vi "E14 BBB Test.vi"(8 "Error In":errorcluster, 10 "Credentials":T1, 11 "SSH Session":refnum<k24>) -> (0 "Error Out":errorcluster, 3 "SSH Session":refnum<k24>)   [LabVIEW 2014, in "LMH-LINX.lvlib"]
uses:
  LMH-LINX.lvlib
  C:/github/makerhub/LINX/LabVIEW/vi.lib/MakerHub/LINX/Private/Utilties/Renci.SshNet.dll
  Renci.SshNet.dll
  <vilib>/MakerHub/Toolbox/LMH-Toolbox.lvlib
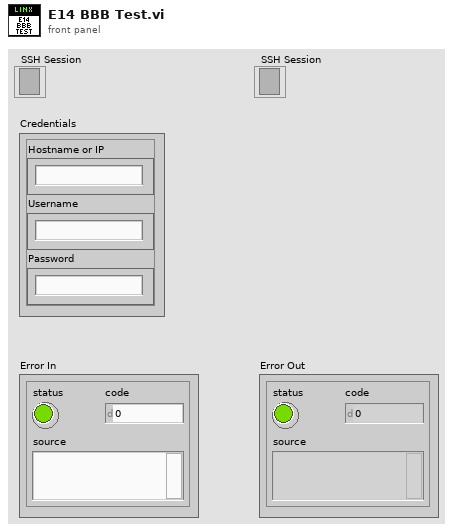
[diagram p1: front panel]
types:
  T1 = cluster{"Hostname or IP":string, "Username":string, "Password":string}
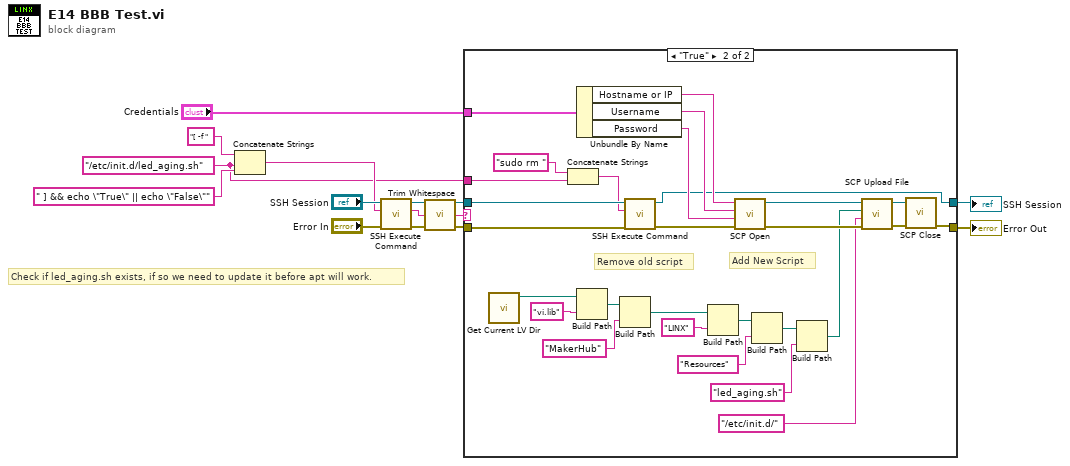
[diagram p0: block diagram]
diagram:
  w6 = "/etc/init.d/led_aging.sh" ("Command")
  # "Check if led_aging.sh exists, if so we need to update it before apt will work."
  n1 = Concatenate Strings("[ -f " ("Command"), w6, " ] && echo \"True\" || echo \"False\"" ("Command")) -> (w7:string)
  n2 = call "SSH Execute Command.vi"("Error In"="Error In", "Command"=w7, "SSH Session"="SSH Session") -> ("Error Out"=w11:errorcluster, "Std Out"=w3:string, "SSH Session"=w10:refnum<k24>)  [unwired: 6 in]
  n3 = call <vilib>:"Trim Whitespace.vi"("string"=w3) -> ("trimmed string"=w2:string)  [unwired: 1 in]
  n4 = case shown="\"True\"" w2 {
    tunnel: w11 -> [w14 w43]
    tunnel: w10 -> [w15 w42]
    tunnel: w6 -> [_ w39]
    tunnel: [w15 w17] -> w4
    tunnel: [w14 w16] -> w5
    tunnel: "Credentials" -> [_ w38]
    frame "False", Default {
      # "Nothing to do here..."
    }
    frame "True" {
      # "Remove old script"
      # "Add New Script"
      n5 = call <vilib>:"Get Current LV Dir.vi"() -> ("This LV Directory"=w22:path)  [unwired: 10 in, 1 out]
      n6 = Concatenate Strings("sudo rm " ("Command"), w39) -> (w40:string)
      n7 = Unbundle By Name(w38) -> ("Hostname or IP"=w37:string, "Username"=w36:string, "Password"=w34:string)
      n8 = Build Path(base path=w22, name or relative path="vi.lib" ("Command")) -> (appended path=w24:path)
      n9 = Build Path(base path=w24, name or relative path="MakerHub" ("Command")) -> (appended path=w25:path)
      n10 = call "SSH Execute Command.vi"("Error In"=w43, "Command"=w40, "SSH Session"=w42) -> ("Error Out"=w35:errorcluster, "SSH Session"=w17:refnum<k24>)  [unwired: 6 in, 1 out]
      n11 = Build Path(base path=w25, name or relative path="LINX" ("Command")) -> (appended path=w26:path)
      n12 = call "SCP Open.vi"("Error In"=w35, "Password"=w34, "Username"=w36, "Hostname or IP"=w37) -> ("Error Out"=w32:errorcluster, "SCP Session"=w33:refnum<k24>)  [unwired: 5 in, 1 out]
      n13 = Build Path(base path=w26, name or relative path="Resources" ("Command")) -> (appended path=w31:path)
      n14 = Build Path(base path=w31, name or relative path="led_aging.sh") -> (appended path=w21:path)
      n15 = call "SCP Upload File.vi"("Error In"=w32, "Target Directory"="/etc/init.d/", "Local File"=w21, "SCP SEssion"=w33) -> ("Error Out"=w19:errorcluster, "SCP Session"=w20:refnum<k24>)  [unwired: 6 in]
      n16 = call "SCP Close.vi"("Error In"=w19, "SCP Session"=w20) -> ("Error Out"=w16:errorcluster)  [unwired: 9 in]
    }
  }
  "Error Out" <- w5
  "SSH Session" <- w4
